vi "Read Commands.vi"(8 "error in (no error)":errorcluster, 11 "CommandDirector in":refnum<class "CommandDirector.lvclass">) -> (0 "error out":errorcluster, 2 "Commands":refnum<class "WriteCommand.lvclass">[](array[class]), 3 "CommandDirector out":refnum<class "CommandDirector.lvclass">)   [LabVIEW 2023, in "HAF.lvlib" / "CommandDirector.lvclass"]
doc: "Returns the current set of Commands operated over."
uses:
  CommandDirector.lvclass
  CommandDirector.lvclass/CommandDirector.ctl
  WriteCommand/WriteCommand.lvclass
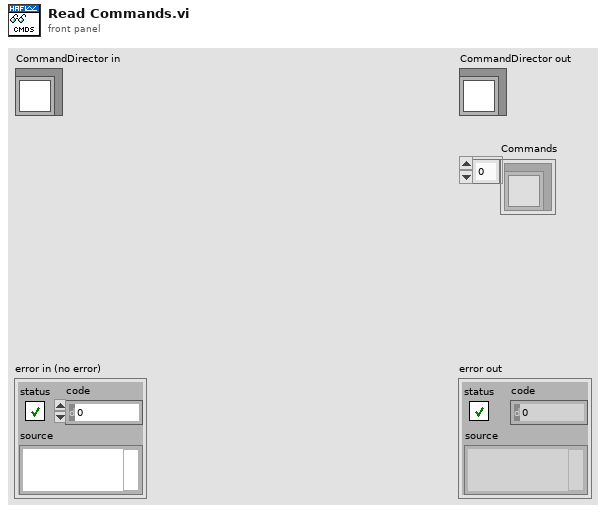
[diagram p1: front panel]
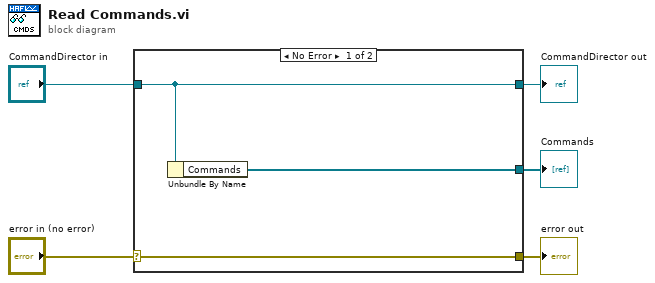
[diagram p0: block diagram]
diagram:
  n1 = case shown="No Error" "error in (no error)" {
    selector: "error in (no error)" -> [w8 w9]
    tunnel: [w8 w9] -> w4
    tunnel: [w7 w10] -> w2
    tunnel: "CommandDirector in" -> [w7 w10]
    tunnel: [w6 _] -> w1
    frame No Error {
      n2 = Unbundle By Name(w7) -> ("Commands"=w6:refnum<class "WriteCommand.lvclass">[])
    }
    frame Error {
    }
  }
  "error out" <- w4
  "CommandDirector out" <- w2
  "Commands" <- w1
